vi "updateK5.vi"(8 "error in (no error)":errorcluster, 11 "reference in":refnum<class "Devices Controller.lvclass">) -> (0 "error out":errorcluster, 3 "reference out":refnum<class "Devices Controller.lvclass">)   [LabVIEW 2016, in "Devices Controller.lvclass"]
uses:
  Devices Controller.lvclass
  deviceType.ctl
  APP/k5_class/k5.lvclass
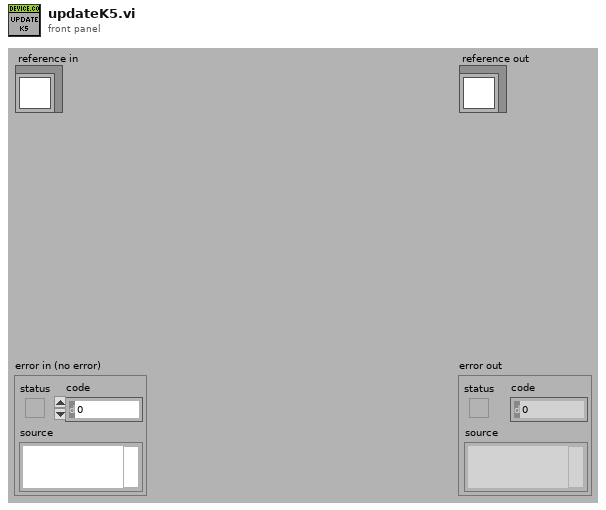
[diagram p1: front panel]
types:
  T1 = typedef "Devices Controller.lvclass/deviceType.ctl" = enum16{"k5", "k4b2", "fitmate", "cpet", "rmr", "bodyBoxPft", "bp", "pp"}
  T2 = cluster{"deviceType":T1, "S/N":string, "SW":string, "Description":string, "Account":string, "System's Location":string, "End User":string, "Email":string, "City":string, "LastChange":string, "Service By":string, "Exp Date":string, "FollowUp Sent":string, "FollowUp Accepted":string, "Note":string}
  T3 = typedef "Devices Controller.lvclass/ObjectAttributesRef.ctl" = refnum<data-value>
  T4 = typedef "Devices Controller.lvclass/ObjectAttributes.ctl" = cluster{"MyAttribute":dbl, "file_controller_ref":refnum<class "File Controller.lvclass">, "data":string[][][], "devices_refs":cluster{"k4b2_refs":refnum<class "k4b2.lvclass">[], "rmr_refs":refnum<class "rmr.lvclass">[], "bod_pod_refs":refnum<class "bodpod.lvclass">[], "cpet_refs":refnum<class "cpet.lvclass">[], "fitmate_refs":refnum<class "fitmate.lvclass">[], "pea_pod_refs":refnum<class "peapod.lvclass">[], "k5_refs":refnum<class "k5.lvclass">[], "bb-pft_refs":refnum<class "bb-pft.lvclass">[]}}
  T5 = cluster{"data[0]":string, "data[1]":string, "data[2]":string, "data[3]":string, "data[4]":string, "data[5]":string, "data[6]":string, "data[7]":string, "data[8]":string}
  T6 = cluster{"[0]":string, "[1]":string, "[2]":string, "[3]":string, "[4]":string, "[5]":string, "[6]":string, "[7]":string, "[8]":string}
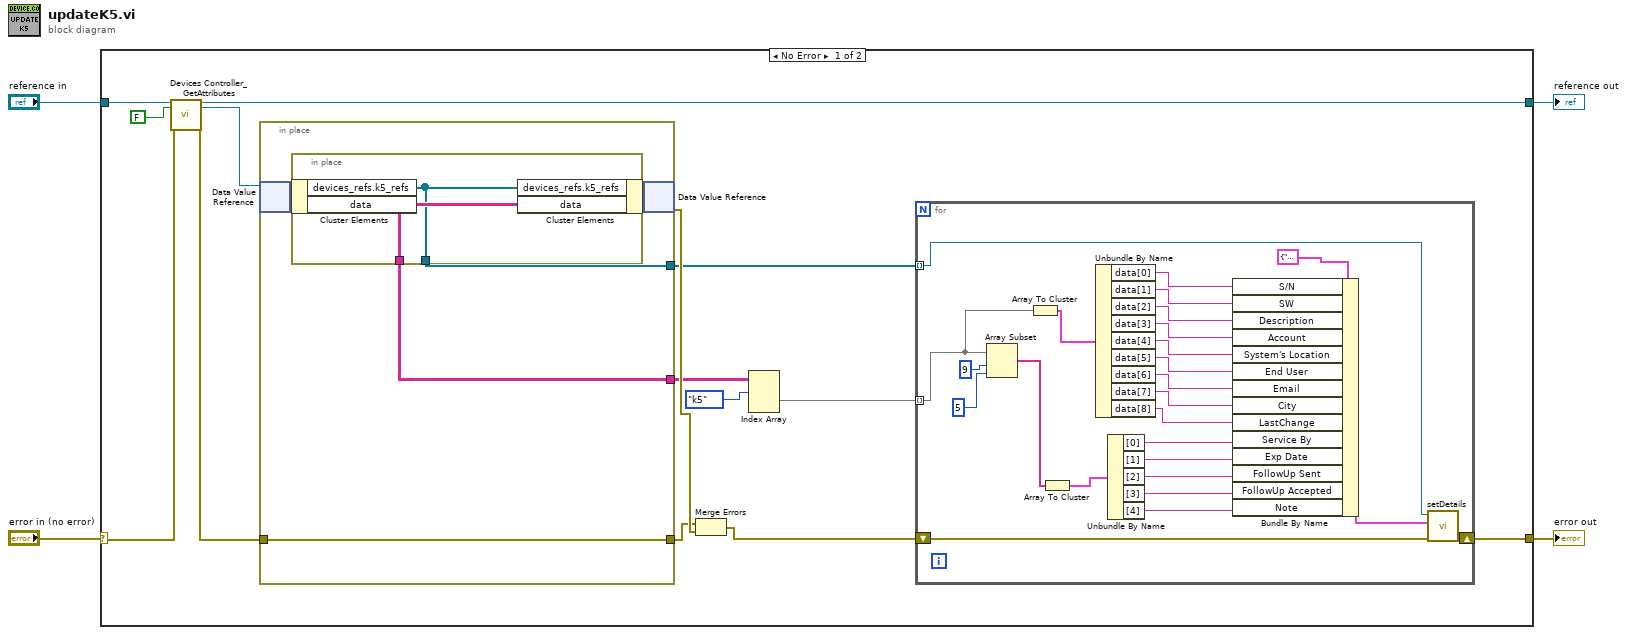
[diagram p0: block diagram]
diagram:
  n1 = case shown="No Error" "error in (no error)" {
    selector: "error in (no error)" -> [w14 w52]
    tunnel: [w9 w52] -> w3
    tunnel: [w12 w51] -> w1
    tunnel: "reference in" -> [w16 w51]
    frame No Error {
      n2 = call "Devices Controller_GetAttributes.vi"("reference in"=w16, "return data? (T)"=FALSE, "error in (no error)"=w14) -> ("reference out"=w12:refnum<class "Devices Controller.lvclass">, "attributes ref"=w11:T3, "error out"=w13:errorcluster)  [unwired: 13 in, 1 out]
      n3 = in-place {
        in-place-border: w13 -> [w46]
        in-place-border: [w46] -> w17
        in-place-border: [w45] -> w7
        in-place-border: [w44] -> w8
        n4 = in-place-dvr #1(w11) -> (w47:T4)  [unwired: 1 out]
        n5 = in-place {
          in-place-border: [w50] -> w45
          in-place-border: [w49] -> w44
          n6 = in-place-cluster #2(w47) -> ("devices_refs.k5_refs"=w49:refnum<class "k5.lvclass">[], "data"=w50:string[][][])
          n7 = in-place-cluster #2("devices_refs.k5_refs"=w49, "data"=w50) -> (w48:T4)
        }
        n8 = in-place-dvr #1(w48) -> (w18:errorcluster)  [unwired: 1 out]
      }
      n9 = Merge Errors(w17, w18) -> (w10:errorcluster)
      n10 = Index Array(array=w7, index (dim 0)=deviceType."k5" ("deviceType")) -> (element=w6:string[][])  [unwired: 2 in]
      n11 = for {
        tunnel: w8 -> [w41] mode=indexing
        tunnel: w6 -> [w35] mode=indexing
        shift-right: [w42] -> w9
        shift-left: w10 -> [w43]
        n12 = Array Subset(array=w35, index=9, length=5) -> (w37:string[])
        n13 = Array To Cluster(array=w35) -> (cluster=w40:T5)
        n14 = Array To Cluster(array=w37) -> (cluster=w36:T6)
        n15 = Unbundle By Name(w40) -> ("data[0]"=w34:string, "data[1]"=w33:string, "data[2]"=w32:string, "data[3]"=w31:string, "data[4]"=w30:string, "data[5]"=w29:string, "data[6]"=w28:string, "data[7]"=w27:string, "data[8]"=w26:string)
        n16 = Unbundle By Name(w36) -> ("[0]"=w25:string, "[1]"=w24:string, "[2]"=w23:string, "[3]"=w22:string, "[4]"=w19:string)
        n17 = Bundle By Name(cluster=T2 {"deviceType"=enum."k5", "S/N"="", "SW"="", "Description"="", "Account"="", "System's Location"="", "End User"="", "Email"="", "City"="", "LastChange"="", "Service By"="", "Exp Date"="", "FollowUp Sent"="", "FollowUp Accepted"="", "Note"=""} ("details"), "S/N"=w34, "SW"=w33, "Description"=w32, "Account"=w31, "System's Location"=w30, "End User"=w29, "Email"=w28, "City"=w27, "LastChange"=w26, "Service By"=w25, "Exp Date"=w24, "FollowUp Sent"=w23, "FollowUp Accepted"=w22, "Note"=w19) -> (w20:T2)
        n18 = call "setDetails.vi"("error in (no error)"=w43, "details"=w20, "reference in"=w41) -> ("error out"=w42:errorcluster)  [unwired: 7 in, 1 out]
      }
    }
    frame Error {
    }
  }
  "error out" <- w3
  "reference out" <- w1
